vi "Full Duplex Streaming (Host).vi"() -> ()   [LabVIEW 2013]
doc: "This template is for the Simple NI-USRP Streaming design, a design that shows the basics of streaming data from an NI 294x/295x device. Refer to the block diagram for more information about how to use this template."
uses:
  <vilib>/userdefined/Silver/nirio_resource_slv.ctl
  SubVIs/Start Trigger.ctl
  <vilib>/Utility/error.llb/DialogType.ctl
  SubVIs/Configure Signal (Level).vi
  SubVIs/Write Tx Data (I16 multi).vi
  SubVIs/Fetch Rx Data (CDB WDT).vi
panel:
  in  "tx active antenna":string(combo)="TX1" caption="Tx Active Antenna"
  in  "rx active antenna":string(combo)="RX1" caption="Rx Active Antenna"
  in  "tx start trigger":T1=enum."Immediate" caption="Tx Start Trigger"
  in  "tone frequency":dbl=100000.0 caption="Tone Frequency" format="%#.3pHz"
  out "Generating":bool
  in  "output power":dbl caption="Output Power" format="%#_gdBm"
  in  "tx channel":string(combo)="tx/RF 1" caption="Tx Channel"
  in  "reference frequency source":string(combo)="Internal" caption="Reference Frequency Source"
  in  "rx channel":string(combo)="rx/RF 0" caption="Rx Channel"
  in  "USRP RIO device":T2="RIO0" caption="USRP RIO Device"
  in  "lo frequency":dbl=-1.0 caption="LO Frequency" format="%#.3pHz"
  in  "number of samples is finite":bool=TRUE
  in  "frequency":dbl=2000000000.0 caption="Frequency" format="%#.3pHz"
  in  "sample rate":dbl=10000000.0 caption="Sample Rate" format="%#.3pS/s"
  in  "reference level":dbl caption="Reference Level" format="%#_gdBm"
  in  "rx start trigger":T1=enum."Immediate" caption="Rx Start Trigger"
  in  "tab control":T3(tab)
  out "Power Spectrum":cluster{"f0":dbl, "df":dbl, "magnitude":dbl[]}(graph)
  out "Power Level":dbl[](graph)
  out "I & Q Data":dbl[][](graph)
  in  "number of samples":u32=8192 caption="Number of Samples"
  in  "stop":bool
  # "Full Duplex Streaming"
  # "This template is for the Simple NI-USRP Streaming design, a design that shows the basics of streaming data from an NI 294x/295x device. See the block diagram for more information on how to use this template."
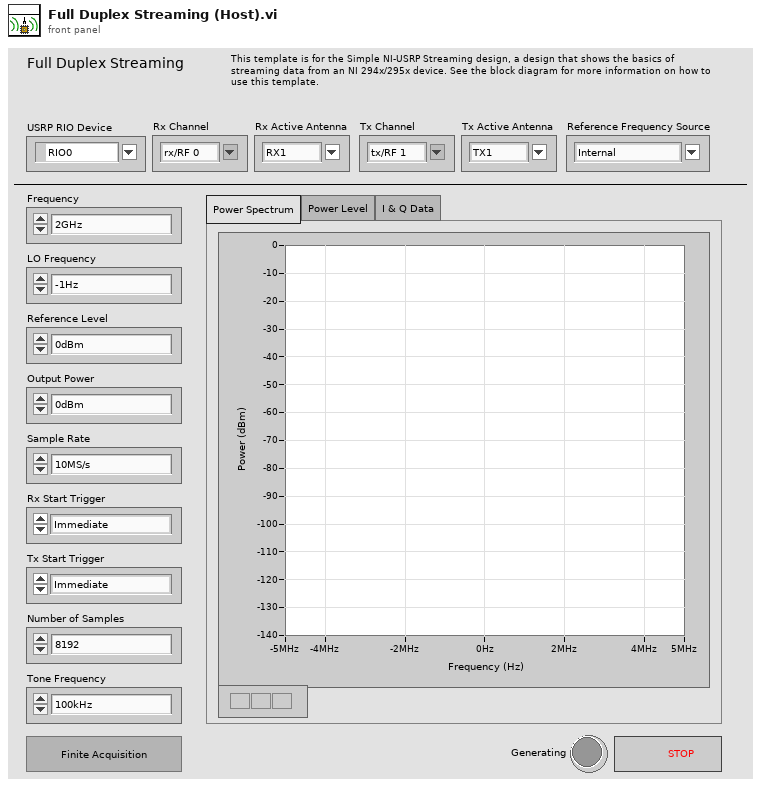
[diagram p1: front panel]
types:
  T1 = typedef "Start Trigger.ctl" = enum8{"Software", "Digital Edge", "Rx Start Trigger", "Tx Start Trigger", "Immediate"}
  T2 = typedef "nirio_resource_slv.ctl" = tag
  T3 = enum32{"Power Spectrum", "Power Level", "I & Q Data"}
  T4 = typedef "DialogType.ctl" = u16
  T5 = typedef "niUsrpRio Config v1 Host.lvlib/niUsrpRio Session.ctl" = cluster{"Global Settings Register Bus":T6, "Radio 0 Settings Register Bus":T6, "Rx NI-USRP session":refnum<k15>, "Tx NI-USRP session":refnum<k15>, "FPGA Interface":refnum<k20>, "RIO Interface Number":u32, "EEPROM Header":T7, "Device Data Header":T8, "EEPROM Characterization Header":T9, "Characterization Data":T10[], "Characterization Data Valid?":bool, "Radio 1 Settings Register Bus":T6, "Radio Settings Bus Semaphore":T12}
  T6 = typedef "niInstr Register Bus v0 Host.lvlib/Register Bus Session.ctl" = refnum<queue>
  T7 = typedef "niUsrpRio Config v1 Host.lvlib/EEPROM Header.ctl" = cluster{"Checksum":u32, "Product Code":u16, "Hardware Current Version":u16, "Hardware Oldest Compatible Version":u16, "EEPROM Map Current Version":u16, "EEPROM Map Oldest Compatible Version":u16, "User Password":string, "Pointer to Factory Header":u32, "Pointer to User Header":u32, "Recommended Interval":u16, "Number of Reserved Bytes":i32, "Number of Daughterboards":u8, "Daughterboard IDs":u16[], "Daughterboard Serial Numbers":string[]}
  T8 = typedef "niUsrpRio Config v1 Host.lvlib/EEPROM Device Data Header.ctl" = cluster{"Checksum":u32, "Number of Channels":u8, "Number of Gain Settings":u16[], "Pointer to Characterization Data":u32[], "Number of Reserved Bytes":i32, "Number of Frequencies":u16[]}
  T9 = typedef "niUsrpRio Config v1 Host.lvlib/EEPROM Characterization Header.ctl" = cluster{"Checksum":u32, "Date":timestamp, "Temperature":sgl, "Misc. Info":string, "Pointer to Device Data Header":u32, "Number of Reserved Bytes":i32}
  T10 = typedef "niUsrpRio Config v1 Host.lvlib/Characterization Data.ctl" = cluster{"Gains[dB]":dbl[], "Frequencies [Hz]":dbl[], "IQ Imbalance Table":T11[], "Measured Gains[dB]":dbl[][]}
  T11 = typedef "niUsrpRio Config v1 Host.lvlib/IQ Imbalance.ctl" = cluster{"Gain Imbalance [linear]":dbl, "Phase Imbalance [radians]":dbl, "Offset":cdb}
  T12 = typedef "Semaphore RefNum" = refnum<k1>
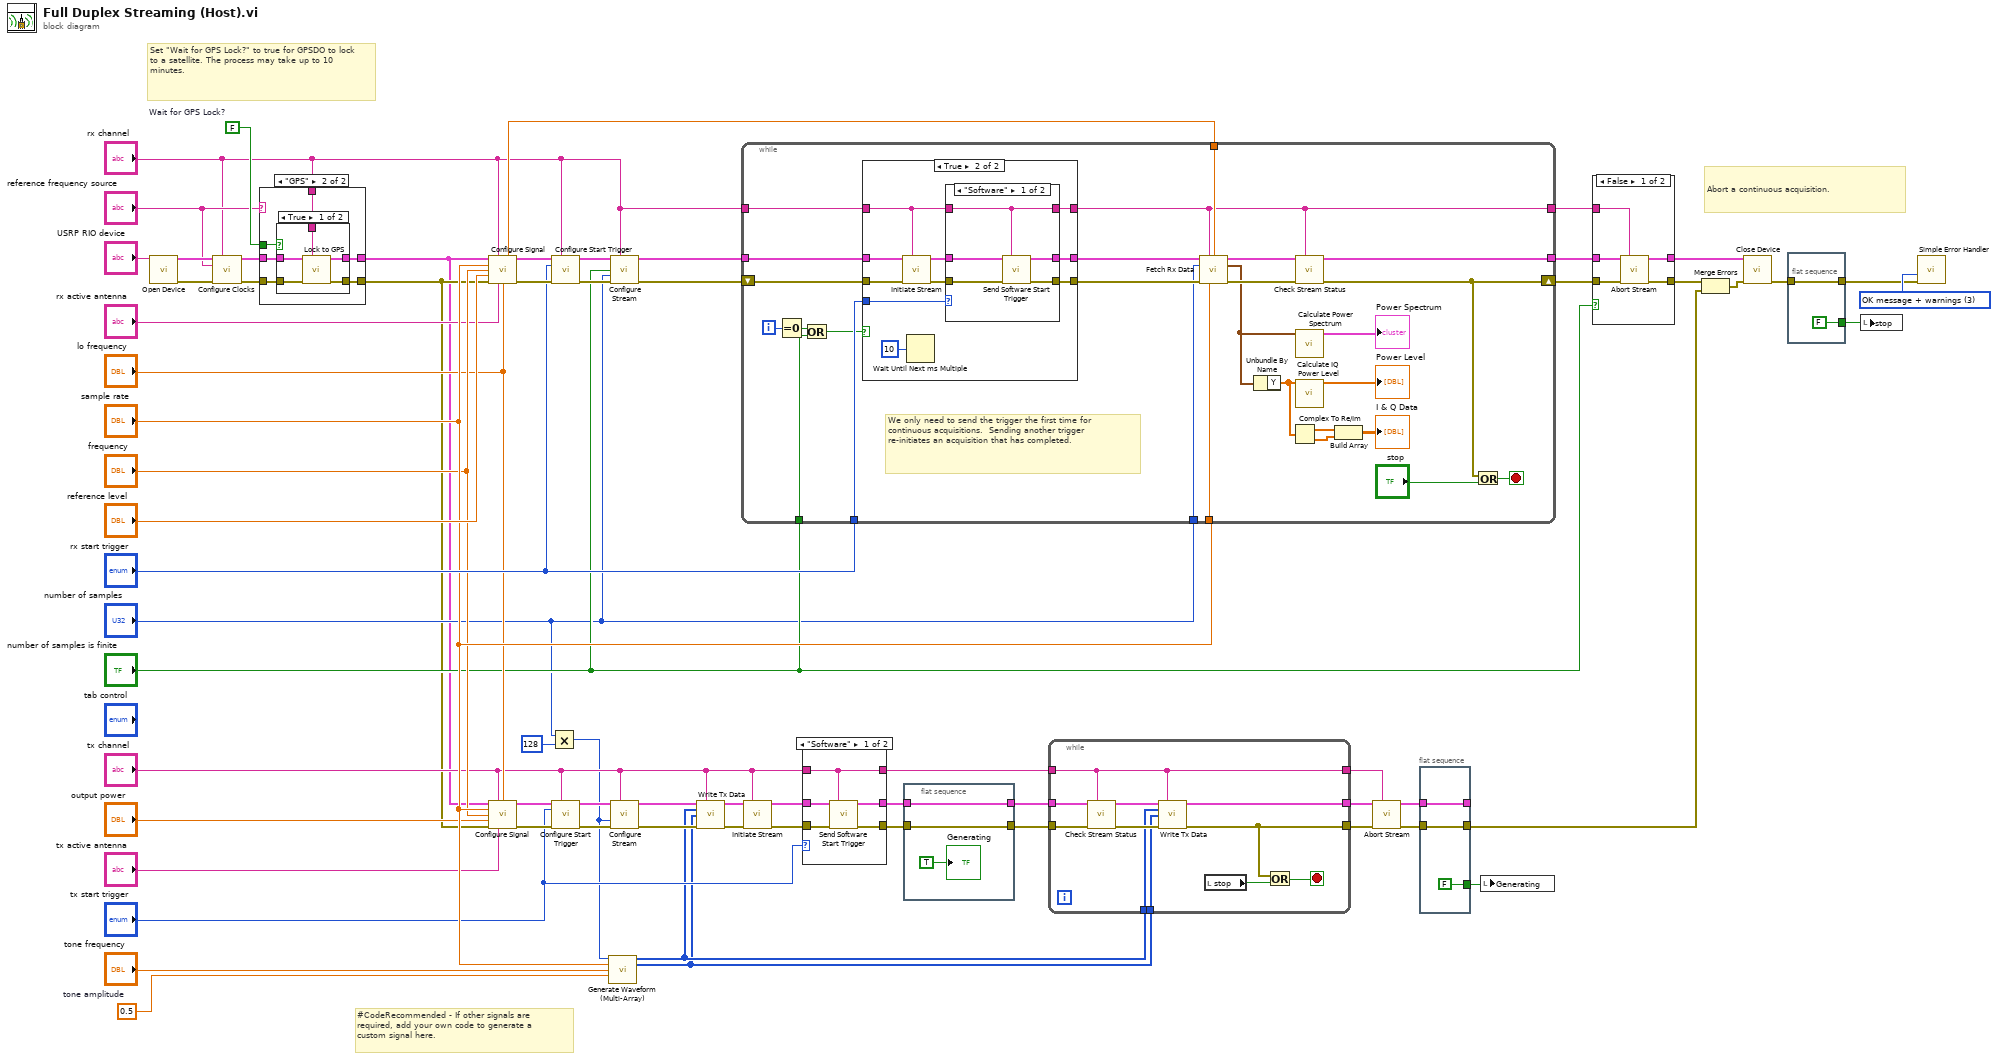
[diagram p0: block diagram]
diagram:
  w1 = 0.5  # tone amplitude
  w10 = FALSE  # Wait for GPS Lock?
  w62 = T4 3 items=["no dialog", "OK message", "continue or stop message", "OK message + warnings", "continue/stop + warnings"] ("type of dialog (OK msg:1)")
  # "Set \"Wait for GPS Lock?\" to true for GPSDO to lock to a satellite. The process may take up to 10 minutes."
  # "#CodeRecommended - If other signals are required, add your own code to generate a custom signal here."
  # "Abort a continuous acquisition."
  n1 = call "Open Device.vi"("USRP RIO device"="USRP RIO device") -> ("niUsrpRio Session (out)"=w4:T5, "error out"=w5:errorcluster)  [unwired: 13 in]
  n2 = call "Configure Clocks.vi"("niUsrpRio Session"=w4, "scope"="rx channel", "Reference Frequency Source"="reference frequency source", "error in"=w5) -> ("niUsrpRio Session (out)"=w7:T5, "error out"=w8:errorcluster)  [unwired: 10 in]
  n3 = case shown="\"GPS\"" "reference frequency source" {
    tunnel: w7 -> [w69 w75]
    tunnel: [w69 w74] -> w6
    tunnel: [w68 w73] -> w9
    tunnel: w8 -> [w68 w72]
    tunnel: "rx channel" -> [_ w71]
    tunnel: w10 -> [_ w70]
    frame Default {
    }
    frame "GPS" {
      n4 = case shown="True" w70 {
        tunnel: w75 -> [w77 w82]
        tunnel: [w80 w82] -> w74
        tunnel: [w79 w81] -> w73
        tunnel: w72 -> [w76 w81]
        tunnel: w71 -> [w78 _]
        frame True {
          n5 = call "Lock to GPS.vi"("niUsrpRio Session"=w77, "scope"=w78, "error in"=w76) -> ("niUsrpRio Session (out)"=w80:T5, "error out"=w79:errorcluster)  [unwired: 11 in]
        }
        frame False {
        }
      }
    }
  }
  n6 = call-poly "Configure Signal.vi"("niUsrpRio Session"=w6, "scope"="rx channel", "sample rate [S/s]"="sample rate", "frequency [Hz]"="frequency", "level [dBm]"="reference level", "error in"=w9, "Active Antenna"="rx active antenna", "LO frequency [Hz]"="lo frequency") -> ("coerced vertical range [Vpp]"=w57:dbl, "niUsrpRio Session (out)"=w60:T5, "error out"=w63:errorcluster)  [unwired: 1 in, 4 out]
  n7 = call-poly "Configure Signal.vi"("niUsrpRio Session"=w6, "scope"="tx channel", "sample rate [S/s]"="sample rate", "frequency [Hz]"="frequency", "level [dBm]"="output power", "error in"=w9, "Active Antenna"="tx active antenna", "LO frequency [Hz]"="lo frequency") -> ("niUsrpRio Session (out)"=w52:T5, "error out"=w66:errorcluster)  [unwired: 1 in, 5 out]
  n8 = Multiply(x="number of samples", y=u32 128) -> (x*y=w14:u32)
  n9 = call "Configure Start Trigger.vi"("niUsrpRio Session"=w60, "scope"="rx channel", "start trigger"="rx start trigger", "error in"=w63) -> ("niUsrpRio Session (out)"=w59:T5, "error out"=w67:errorcluster)  [unwired: 10 in]
  n10 = call "Configure Start Trigger.vi"("niUsrpRio Session"=w52, "scope"="tx channel", "start trigger"="tx start trigger", "error in"=w66) -> ("niUsrpRio Session (out)"=w51:T5, "error out"=w65:errorcluster)  [unwired: 10 in]
  n11 = call "Generate Waveform (Multi-Array).vi"("number of samples"=w14, "sample rate"="sample rate", "tone frequency"="tone frequency", "amplitude"=w1) -> ("I"=w17:i16[], "Q"=w16:i16[])  [unwired: 9 in, 1 out]
  n12 = call "Configure Stream.vi"("niUsrpRio Session"=w59, "scope"="rx channel", "number of samples is finite"="number of samples is finite", "number of samples"="number of samples", "error in"=w67) -> ("niUsrpRio Session (out)"=w33:T5, "error out"=w30:errorcluster)  [unwired: 9 in]
  n13 = call "Configure Stream.vi"("niUsrpRio Session"=w51, "scope"="tx channel", "number of samples"=w14, "error in"=w65) -> ("niUsrpRio Session (out)"=w50:T5, "error out"=w64:errorcluster)  [unwired: 10 in]
  n14 = call-poly "Write Tx Data.vi"("niUsrpRio Session"=w50, "scope"="tx channel", "I"=w17, "Q"=w16, "error in"=w64) -> ("niUsrpRio Session (out)"=w21:T5, "error out"=w22:errorcluster)  [unwired: 9 in]
  n15 = while {
    tunnel: w33 -> [w99]
    tunnel: [w107] -> w56
    tunnel: w57 -> [w91]
    tunnel: "sample rate" -> [w90]
    tunnel: "number of samples" -> [w89]
    tunnel: "rx start trigger" -> [w102]
    tunnel: "number of samples is finite" -> [w86]
    shift-right: [w106] -> w55
    shift-left: w30 -> [w101]
    tunnel: "rx channel" -> [w84]
    tunnel: [w83] -> w11
    i -> [w87]
    stop <- w109 stop-if-true
    # "We only need to send the trigger the first time for continuous acquisitions.  Sending another trigger re-initiates an acquisition that has completed."
    # "Acquire and Fetch a waveform"
    n16 = Equal To 0?(x=w87) -> (x = 0?=w88:bool)
    n17 = Or(x=w88, y=w86) -> (x .or. y?=w85:bool)
    n18 = case shown="True" w85 {
      tunnel: w102 -> [_ w122]
      tunnel: w101 -> [w111 w117]
      tunnel: [w111 w121] -> w100
      tunnel: w99 -> [w112 w119]
      tunnel: [w112 w120] -> w98
      tunnel: w84 -> [w110 w115]
      tunnel: [w110 w114] -> w83
      frame False {
      }
      frame True {
        n19 = call "Initiate Stream.vi"("niUsrpRio Session"=w119, "scope"=w115, "error in"=w117) -> ("niUsrpRio Session (out)"=w118:T5, "error out"=w116:errorcluster)  [unwired: 11 in]
        n20 = Wait Until Next ms Multiple(millisecond multiple=u32 10) -> ()  [unwired: 1 out]
        n21 = case shown="\"Software\"" w122 {
          tunnel: w116 -> [w127 w130]
          tunnel: w118 -> [w125 w129]
          tunnel: [w126 w130] -> w121
          tunnel: [w124 w129] -> w120
          tunnel: w115 -> [w123 w128]
          tunnel: [w123 w128] -> w114
          frame "Software" {
            # "Send the software trigger to the master device only.  The master will also trigger all slave devices."
            n22 = call "Send Software Start Trigger.vi"("niUsrpRio Session"=w125, "scope"=w123, "error in"=w127) -> ("niUsrpRio Session (out)"=w124:T5, "error out"=w126:errorcluster)  [unwired: 11 in]
          }
          frame Default {
          }
        }
      }
    }
    n23 = call-poly "Fetch Rx Data.vi"("niUsrpRio Session"=w98, "scope"=w83, "vertical range [Vpp]"=w91, "number of samples"=w89, "error in"=w100, "sample rate"=w90) -> ("niUsrpRio Session (out)"=w92:T5, "Waveform (CDB WDT)"=w95:waveform(cdb), "error out"=w97:errorcluster)  [unwired: 7 in]
    n24 = Unbundle By Name(w95) -> ("Y"=w96:cdb[])
    n25 = Complex To Re/Im(x + iy=w96) -> (x=w94:dbl[], y=w93:dbl[])
    n26 = call "Check Stream Status.vi"("niUsrpRio Session"=w92, "scope"=w83, "error in"=w97) -> ("niUsrpRio Session (out)"=w107:T5, "error out"=w106:errorcluster)  [unwired: 10 in, 1 out]
    n27 = call "Calculate Power Spectrum.vi"("IQ Waveform"=w95) -> ("power spectrum (dBm)"=→"Power Spectrum":cluster{"f0":dbl, "df":dbl, "magnitude":dbl[]})  [unwired: 14 in]
    n28 = call "Calculate IQ Power Level.vi"("IQ data"=w96) -> ("power level (dBm)"=→"Power Level":dbl[])  [unwired: 14 in]
    n29 = Build Array(w94, w93) -> (→"I & Q Data":dbl[][])
    n30 = Or(x=w106, y="stop") -> (x .or. y?=w109:bool)
  }
  n31 = call "Initiate Stream.vi"("niUsrpRio Session"=w21, "scope"="tx channel", "error in"=w22) -> ("niUsrpRio Session (out)"=w28:T5, "error out"=w23:errorcluster)  [unwired: 11 in]
  n32 = case shown="\"Software\"" "tx start trigger" {
    tunnel: w23 -> [w135 w138]
    tunnel: w28 -> [w133 w137]
    tunnel: [w134 w138] -> w26
    tunnel: [w132 w137] -> w27
    tunnel: "tx channel" -> [w131 w136]
    tunnel: [w131 w136] -> w18
    frame "Software" {
      # "Send the software trigger to the master device only.  The master will also trigger all slave devices."
      n33 = call "Send Software Start Trigger.vi"("niUsrpRio Session"=w133, "scope"=w131, "error in"=w135) -> ("niUsrpRio Session (out)"=w132:T5, "error out"=w134:errorcluster)  [unwired: 11 in]
    }
    frame Default {
    }
  }
  n34 = flat-sequence {
    tunnel: w27 -> [w141]
    tunnel: w26 -> [w140]
    tunnel: [w141] -> w25
    tunnel: [w140] -> w24
    frame #0 {
      "Generating" <- TRUE ("Generating")
    }
  }
  n35 = while {
    tunnel: w25 -> [w152]
    tunnel: w24 -> [w151]
    tunnel: [w147] -> w20
    tunnel: [w146] -> w19
    tunnel: w18 -> [w143]
    tunnel: w17 -> [w145]
    tunnel: w16 -> [w144]
    tunnel: [w143] -> w15
    stop <- w142 stop-if-true
    n36 = call "Check Stream Status.vi"("niUsrpRio Session"=w152, "scope"=w143, "error in"=w151) -> ("niUsrpRio Session (out)"=w149:T5, "error out"=w148:errorcluster)  [unwired: 10 in, 1 out]
    n37 = call-poly "Write Tx Data.vi"("niUsrpRio Session"=w149, "scope"=w143, "I"=w145, "Q"=w144, "error in"=w148) -> ("niUsrpRio Session (out)"=w146:T5, "error out"=w147:errorcluster)  [unwired: 9 in]
    n38 = local read "stop"() -> (w150:bool)
    n39 = Or(x=w147, y=w150) -> (x .or. y?=w142:bool)
  }
  n40 = call "Abort Stream.vi"("niUsrpRio Session"=w19, "scope"=w15, "error in"=w20) -> ("niUsrpRio Session (out)"=w41:T5, "error out"=w42:errorcluster)  [unwired: 11 in]
  n41 = flat-sequence {
    tunnel: [w155] -> _
    tunnel: w41 -> [w155]
    tunnel: [w154] -> w37
    tunnel: w42 -> [w154]
    tunnel: [FALSE ("Generating")] -> w40
    frame #0 {
    }
  }
  n42 = local write "Generating"(w40) -> ()
  n43 = case shown="False" "number of samples is finite" {
    tunnel: w56 -> [w160 w162]
    tunnel: w55 -> [w159 w161]
    tunnel: [w158 w162] -> w54
    tunnel: [w157 w161] -> w39
    tunnel: w11 -> [w156 _]
    frame False {
      n44 = call "Abort Stream.vi"("niUsrpRio Session"=w160, "scope"=w156, "error in"=w159) -> ("niUsrpRio Session (out)"=w158:T5, "error out"=w157:errorcluster)  [unwired: 11 in]
    }
    frame True {
    }
  }
  n45 = Merge Errors(w39, w37) -> (w38:errorcluster)
  n46 = call "Close Device.vi"("niUsrpRio Session"=w54, "error in"=w38) -> ("error out"=w36:errorcluster)  [unwired: 13 in]
  n47 = flat-sequence {
    tunnel: w36 -> [w164]
    tunnel: [w164] -> w35
    tunnel: [FALSE] -> w34
    frame #0 {
    }
  }
  n48 = local write "stop"(w34) -> ()
  n49 = call <vilib>:"Simple Error Handler.vi"("type of dialog (OK msg:1)"=w62, "error in (no error)"=w35) -> ()  [unwired: 3 in, 5 out]
